vi "获取二维数组值.vi"(1 "索引":i32, 2 "数组":i32[][](array[numeric])) -> (0 "数值":i32)   [LabVIEW 2017]
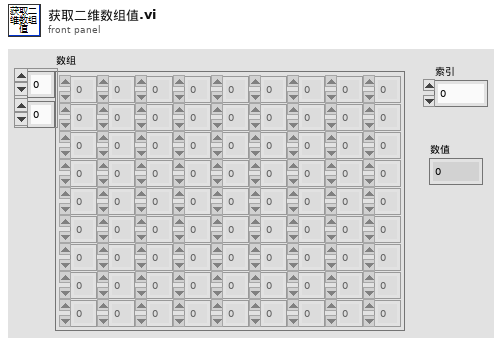
[diagram p1: front panel]
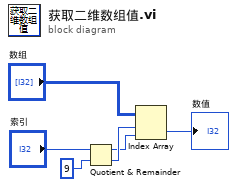
[diagram p0: block diagram]
diagram:
  n1 = Quotient & Remainder(x="索引", y=9) -> (x-y*floor(x/y)=w3:i32, floor(x/y)=w4:i32)
  n2 = Index Array(array="数组", index (row)=w4, index (col)=w3) -> (element=→"数值":i32)
